vi "Array Sizer.vi"(2 "maxV":dbl=20.0 step=5.0, 3 "turn accel":dbl, 4 "Overrides":T1 {"Angle Override" step=5.0; "Velocity Override" step=5.0; "Angular Override" step=5.0}, 5 "Points out":cluster{"x":dbl, "y":dbl, "th":dbl}[](array[cluster])) -> (1 "Overrides out":T1 {"Angle Override" step=5.0; "Velocity Override" step=5.0; "Angular Override" step=5.0})   [LabVIEW 2025]
uses:
  Types/Overrides.ctl
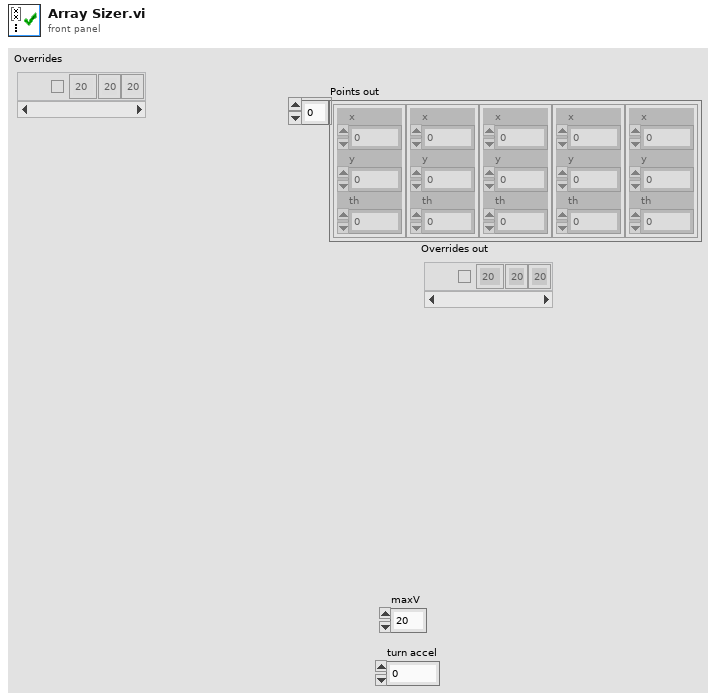
[diagram p1: front panel]
types:
  T1 = typedef "Overrides.ctl" = cluster{"Count":string, "Angular Override":dbl, "Enabled?":bool, "Velocity Override":dbl, "Angle Override":dbl}[]
  T2 = cluster{"Count":string, "Angular Override":dbl, "Enabled?":bool, "Velocity Override":dbl, "Angle Override":dbl}
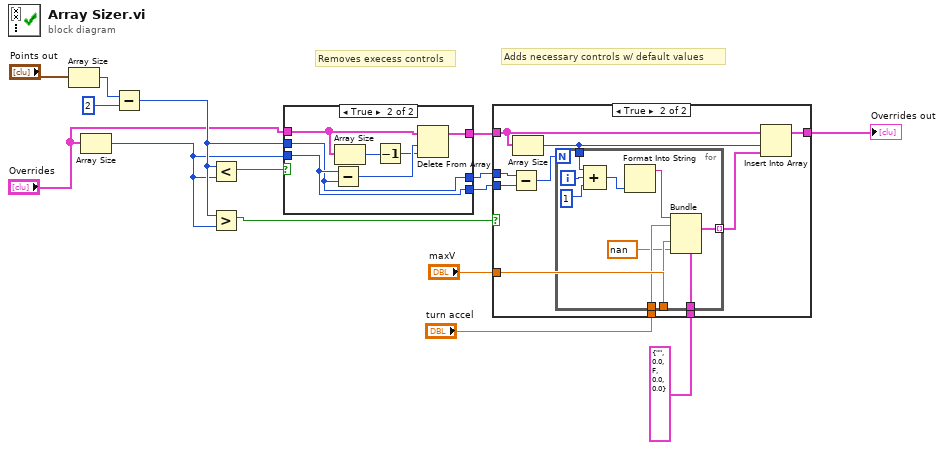
[diagram p0: block diagram]
diagram:
  # "Adds necessary controls w/ default values"
  # "Removes execess controls"
  n1 = Array Size(array="Points out") -> (size(s)=w15:i32)
  n2 = Array Size(array="Overrides") -> (size(s)=w10:i32)
  n3 = Subtract(x=w15, y=2) -> (x-y=w11:i32)
  n4 = Less?(x=w11, y=w10) -> (x < y?=w12:bool)
  n5 = Greater?(x=w11, y=w10) -> (0:w6:bool)
  n6 = case shown="True" w12 {
    tunnel: [w18 w19] -> w9
    tunnel: "Overrides" -> [w18 w22]
    tunnel: w11 -> [w17 w24]
    tunnel: w10 -> [w16 w25]
    tunnel: [w17 w24] -> w8
    tunnel: [w16 w25] -> w7
    frame False {
    }
    frame True {
      n7 = Subtract(x=w25, y=w24) -> (x-y=w23:i32)
      n8 = Array Size(array=w22) -> (size(s)=w21:i32)
      n9 = Decrement(x=w21) -> (x-1=w20:i32)
      n10 = Delete From Array(array=w22, length=w23, index=w20) -> (array with subset deleted=w19:T1)  [unwired: 1 out]
    }
  }
  n11 = case shown="True" w6 {
    tunnel: [w26 w33] -> w2
    tunnel: w9 -> [w26 w28]
    tunnel: w8 -> [_ w36]
    tunnel: w7 -> [_ w35]
    tunnel: "maxV" -> [_ w31]
    tunnel: "turn accel" -> [_ w29]
    tunnel: T2 {"Count"="", "Angular Override"=0.0, "Enabled?"=FALSE, "Velocity Override"=0.0, "Angle Override"=0.0} ("output cluster") -> [_ w27]
    frame False {
    }
    frame True {
      n12 = Subtract(x=w36, y=w35) -> (x-y=w34:i32)
      n13 = Array Size(array=w28) -> (size(s)=w30:i32)
      n14 = for {
        N: w34 -> [_]
        tunnel: [w45] -> w32 mode=indexing
        tunnel: w31 -> [w46]
        tunnel: w30 -> [w43]
        tunnel: w29 -> [w39]
        tunnel: w27 -> [w37]
        i -> [w44]
        n15 = Compound Arithmetic op=ADD(w43, w44, 1) -> (w42:i32)
        n16 = Format Into String(w42) -> (resulting string=w41:string)  [unwired: 3 in, 1 out]
        n17 = Bundle(cluster=w37, "Count"=w41, "Angular Override"=w39, "Velocity Override"=w46, "Angle Override"=nan) -> (w45:T2)  [unwired: 1 in]
      }
      n18 = Insert Into Array(array=w28, index=w30, new element=w32) -> (w33:T1)
    }
  }
  "Overrides out" <- w2
